vi "writeValue.vi"(8 "error in (no error)":errorcluster, 9 "Value":dbl format="%_8f", 10 "Sensor":u8, 11 "RTMockDisplacement in":refnum<class "RTMockDisplacement.lvclass">) -> (0 "error out":errorcluster, 3 "RTMockDisplacement out":refnum<class "RTMockDisplacement.lvclass">)   [LabVIEW 2016, in "RTMockDisplacement.lvlib" / "RTMockDisplacement.lvclass"]
uses:
  RTMockDisplacement.lvclass
  RTMockDisplacement.lvclass/RTMockDisplacement.ctl
  Common_RT_FPGA/IWriteU8FIFO/IWriteU8FIFO.lvclass
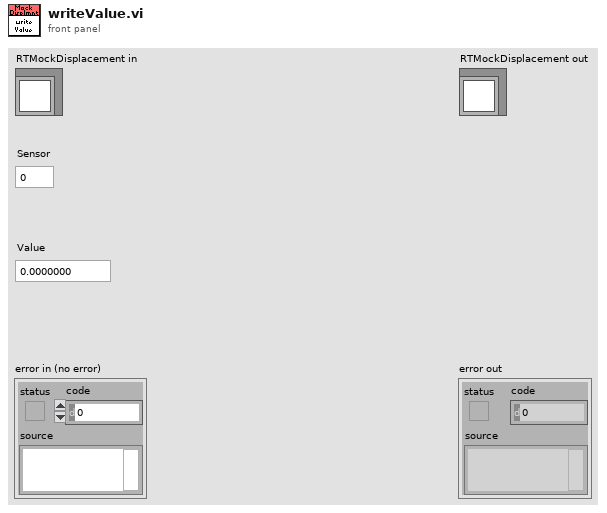
[diagram p1: front panel]
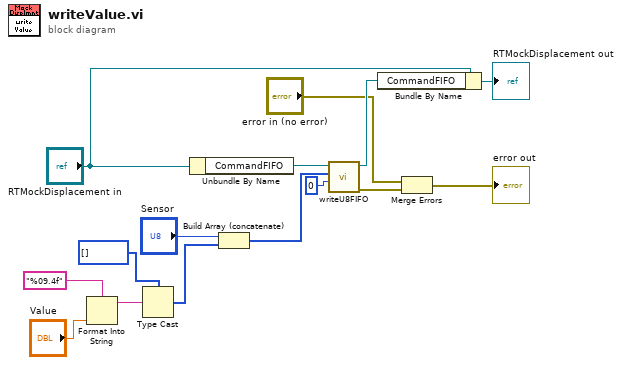
[diagram p0: block diagram]
diagram:
  n1 = Format Into String(format string="%09.4f", "Value") -> (resulting string=w13:string)  [unwired: 2 in, 1 out]
  n2 = Type Cast(type=u8[] [], x=w13) -> (*(type *) &x=w10:u8[])
  n3 = Unbundle By Name("RTMockDisplacement in") -> ("CommandFIFO"=w7:refnum<class "IWriteU8FIFO.lvclass">)
  n4 = Build Array (concatenate)("Sensor", w10) -> (w9:u8[])
  n5 = call-dynamic "writeU8FIFO.vi"("Timeout"=0, "Data"=w9, "IWriteU8FIFO in"=w7) -> ("error out"=w3:errorcluster, "IWriteU8FIFO out"=w6:refnum<class "IWriteU8FIFO.lvclass">)  [unwired: 6 in, 1 out]
  n6 = Bundle By Name(cluster="RTMockDisplacement in", "CommandFIFO"=w6) -> (→"RTMockDisplacement out":refnum<class "RTMockDisplacement.lvclass">)
  n7 = Merge Errors("error in (no error)", w3) -> (→"error out":errorcluster)
